vi "SR_M-Gen_Mission_annotations.vi"(10 "Op Index":i32=-1, 11 "Mission In":T1[](array[typedef]) {"GPS Longitude" format="%.6g"; "GPS Latitude" format="%.6g"}) -> (1 "Mission Path":cluster{dbl[], dbl[]}, 2 "Mission Annotation":T2(array[cluster]), 3 "Mission Out":T1[](array[typedef]) {"GPS Longitude" format="%.6g"; "GPS Latitude" format="%.6g"})   [LabVIEW 2015, in "Shore Library.lvlib"]
uses:
  Shore Library.lvlib
  RDS Mission Controller Actor/MissionOp.ctl
  RDS Mission Controller Actor/RDS Mission Controller Actor.lvlib
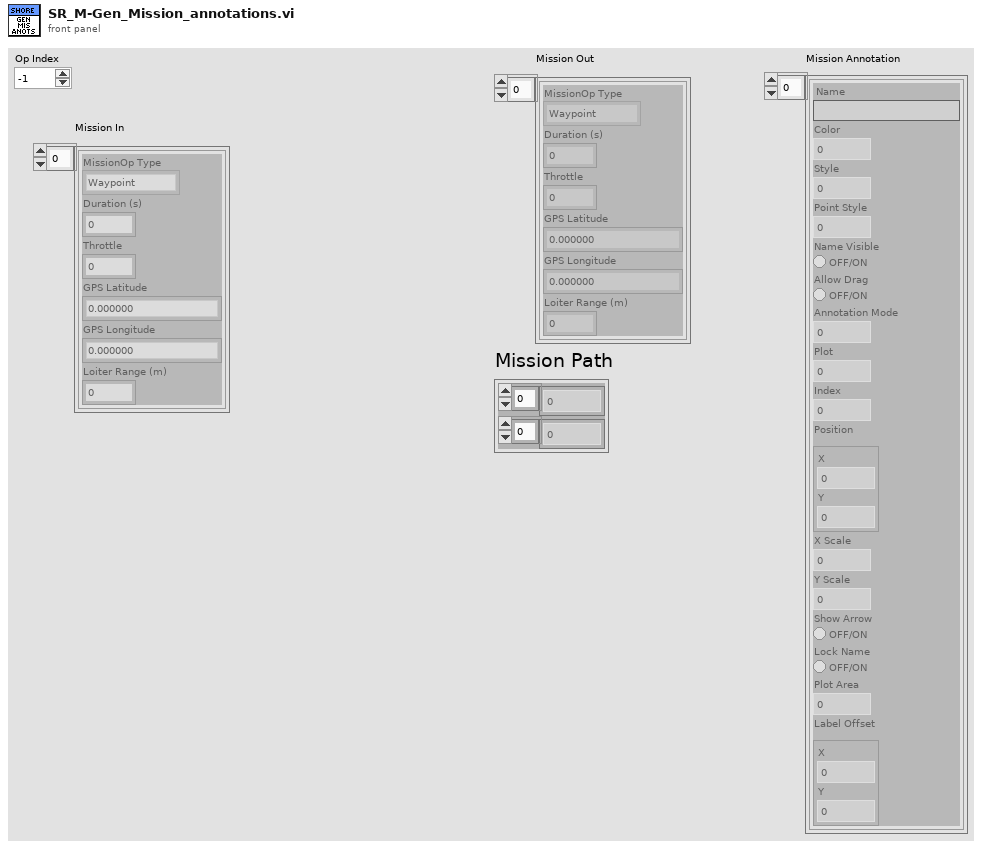
[diagram p1: front panel]
types:
  T1 = typedef "RDS Mission Controller Actor.lvlib/MissionOp.ctl" = cluster{"MissionOp Type":enum16{"Waypoint", "Loiter", "Wait", "Deploy AIP", "Stow AIP"}, "Duration (s)":u16, "Throttle":i16, "GPS Latitude":dbl, "GPS Longitude":dbl, "Loiter Range (m)":u16}
  T2 = cluster{"Name":string, "Color":u32, "Style":u8, "Point Style":u8, "Name Visible":bool, "Allow Drag":bool, "Annotation Mode":u32, "Plot":i32, "Index":i32, "Position":cluster{"X":dbl, "Y":dbl}, "X Scale":u32, "Y Scale":u32, "Show Arrow":bool, "Lock Name":bool, "Plot Area":i32, "Label Offset":cluster{"X":dbl, "Y":dbl}}[]
  T3 = cluster{"Name":string, "Color":u32, "Style":u8, "Point Style":u8, "Name Visible":bool, "Allow Drag":bool, "Annotation Mode":u32, "Plot":i32, "Index":i32, "Position":cluster{"X":dbl, "Y":dbl}, "X Scale":u32, "Y Scale":u32, "Show Arrow":bool, "Lock Name":bool, "Plot Area":i32, "Label Offset":cluster{"X":dbl, "Y":dbl}}
  T4 = enum16{"Waypoint", "Loiter", "Wait", "Deploy AIP", "Stow AIP"}
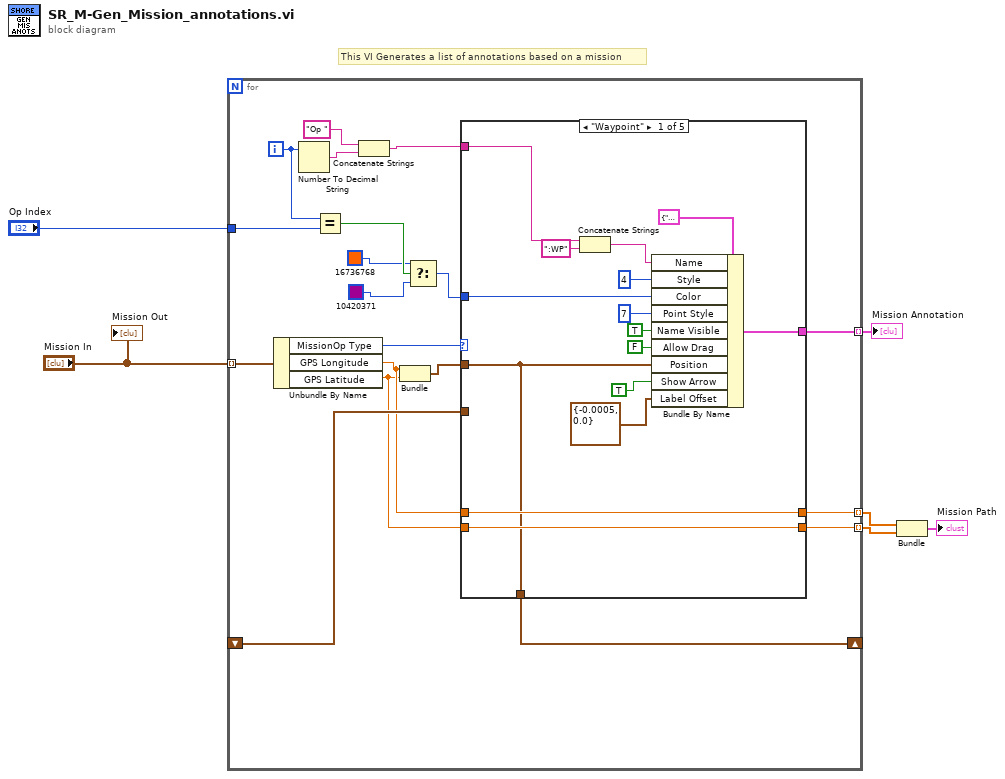
[diagram p0: block diagram]
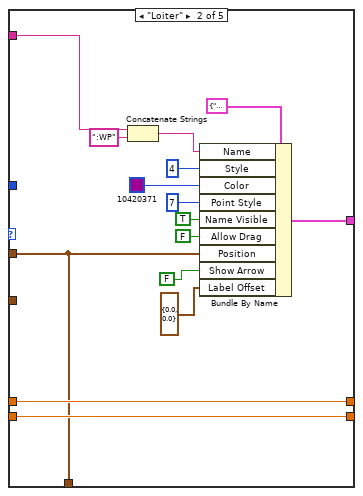
[diagram p2: hidden frame]
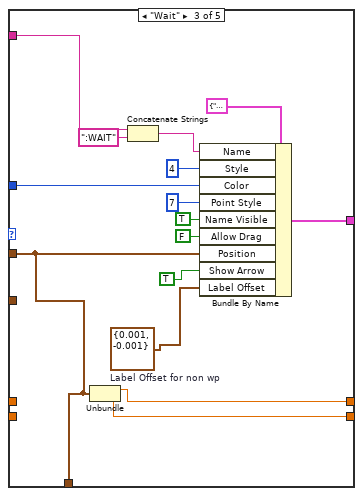
[diagram p3: hidden frame]
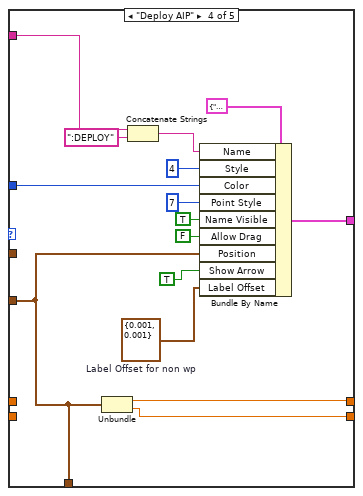
[diagram p4: hidden frame]
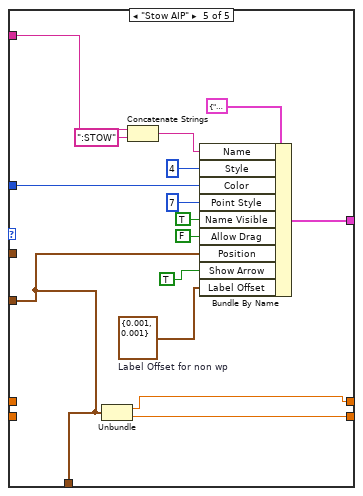
[diagram p5: hidden frame]
diagram:
  # "This VI Generates a list of annotations based on a mission"
  n1 = for {
    tunnel: "Mission In" -> [w20] mode=indexing
    tunnel: [w21] -> w5 mode=indexing
    shift-right: [w7] -> _
    shift-left: _ -> [w19]
    tunnel: "Op Index" -> [w17]
    tunnel: [w10] -> w3 mode=indexing
    tunnel: [w9] -> w2 mode=indexing
    i -> [w18]
    n2 = Unbundle By Name(w20) -> ("MissionOp Type"=w25:T4, "GPS Longitude"=w12:dbl, "GPS Latitude"=w11:dbl)
    n3 = Number To Decimal String(number=w18) -> (decimal integer string=w24:string)  [unwired: 1 in]
    n4 = Equal?(x=w18, y=w17) -> (x = y?=w16:bool)
    n5 = Concatenate Strings("Op " ("string"), w24) -> (w22:string)
    n6 = Bundle("GPS Longitude"=w12, "GPS Latitude"=w11) -> (w8:cluster{"GPS Longitude":dbl, "GPS Latitude":dbl})  [unwired: 1 in]
    n7 = Select(t=u32 16736768 ("Color of Annotation Text"), s=w16, f=u32 10420371 ("Color of Annotation Text")) -> (s? t:f=w14:u32)
    n8 = case shown="\"Waypoint\"" w25 {
      tunnel: w22 -> [w32 w46 w63 w78 w93]
      tunnel: [w33 w47 w64 w79 w94] -> w21
      tunnel: w8 -> [w26 w41 w56 _ _]
      tunnel: w14 -> [w29 _ w60 w75 w90]
      tunnel: w19 -> [_ _ _ w71 w86]
      tunnel: w12 -> [w28 w43 _ _ _]
      tunnel: w11 -> [w27 w42 _ _ _]
      tunnel: [w28 w43 w58 w73 w88] -> w10
      tunnel: [w27 w42 w57 w72 w87] -> w9
      tunnel: [w26 w41 w56 w71 w86] -> w7
      frame "Waypoint" {
        n9 = Concatenate Strings(w32, ":WP" ("string")) -> (w31:string)
        n10 = Bundle By Name(cluster=T3 {"Name"="", "Color"=0, "Style"=0, "Point Style"=0, "Name Visible"=FALSE, "Allow Drag"=FALSE, "Annotation Mode"=0, "Plot"=0, "Index"=0, "Position"={"X"=0.0, "Y"=0.0}, "X Scale"=0, "Y Scale"=0, "Show Arrow"=FALSE, "Lock Name"=FALSE, "Plot Area"=0, "Label Offset"={"X"=0.0, "Y"=0.0}}, "Name"=w31, "Style"=u8 4, "Color"=w29, "Point Style"=u8 7, "Name Visible"=TRUE, "Allow Drag"=FALSE, "Position"=w26, "Show Arrow"=TRUE, "Label Offset"=cluster{"X":dbl, "Y":dbl} {"X"=-0.0005, "Y"=0.0}) -> (w33:T3)
      }
      frame "Loiter" {
        n11 = Concatenate Strings(w46, ":WP" ("string")) -> (w45:string)
        n12 = Bundle By Name(cluster=T3 {"Name"="", "Color"=0, "Style"=0, "Point Style"=0, "Name Visible"=FALSE, "Allow Drag"=FALSE, "Annotation Mode"=0, "Plot"=0, "Index"=0, "Position"={"X"=0.0, "Y"=0.0}, "X Scale"=0, "Y Scale"=0, "Show Arrow"=FALSE, "Lock Name"=FALSE, "Plot Area"=0, "Label Offset"={"X"=0.0, "Y"=0.0}}, "Name"=w45, "Style"=u8 4, "Color"=u32 10420371 ("Color of Annotation Text"), "Point Style"=u8 7, "Name Visible"=TRUE, "Allow Drag"=FALSE, "Position"=w41, "Show Arrow"=FALSE, "Label Offset"=cluster{"X":dbl, "Y":dbl} {"X"=0.0, "Y"=0.0}) -> (w47:T3)
      }
      frame "Wait" {
        w59 = cluster{"X":dbl, "Y":dbl} {"X"=0.001, "Y"=-0.001}  # Label Offset for non wp
        n13 = Unbundle(w56) -> ("GPS Longitude"=w58:dbl, "GPS Latitude"=w57:dbl)
        n14 = Concatenate Strings(w63, ":WAIT" ("string")) -> (w62:string)
        n15 = Bundle By Name(cluster=T3 {"Name"="", "Color"=0, "Style"=0, "Point Style"=0, "Name Visible"=FALSE, "Allow Drag"=FALSE, "Annotation Mode"=0, "Plot"=0, "Index"=0, "Position"={"X"=0.0, "Y"=0.0}, "X Scale"=0, "Y Scale"=0, "Show Arrow"=FALSE, "Lock Name"=FALSE, "Plot Area"=0, "Label Offset"={"X"=0.0, "Y"=0.0}}, "Name"=w62, "Style"=u8 4, "Color"=w60, "Point Style"=u8 7, "Name Visible"=TRUE, "Allow Drag"=FALSE, "Position"=w56, "Show Arrow"=TRUE, "Label Offset"=w59) -> (w64:T3)
      }
      frame "Deploy AIP" {
        w74 = cluster{"X":dbl, "Y":dbl} {"X"=0.001, "Y"=0.001}  # Label Offset for non wp
        n16 = Unbundle(w71) -> ("GPS Longitude"=w73:dbl, "GPS Latitude"=w72:dbl)
        n17 = Concatenate Strings(w78, ":DEPLOY" ("string")) -> (w77:string)
        n18 = Bundle By Name(cluster=T3 {"Name"="", "Color"=0, "Style"=0, "Point Style"=0, "Name Visible"=FALSE, "Allow Drag"=FALSE, "Annotation Mode"=0, "Plot"=0, "Index"=0, "Position"={"X"=0.0, "Y"=0.0}, "X Scale"=0, "Y Scale"=0, "Show Arrow"=FALSE, "Lock Name"=FALSE, "Plot Area"=0, "Label Offset"={"X"=0.0, "Y"=0.0}}, "Name"=w77, "Style"=u8 4, "Color"=w75, "Point Style"=u8 7, "Name Visible"=TRUE, "Allow Drag"=FALSE, "Position"=w71, "Show Arrow"=TRUE, "Label Offset"=w74) -> (w79:T3)
      }
      frame "Stow AIP" {
        w89 = cluster{"X":dbl, "Y":dbl} {"X"=0.001, "Y"=0.001}  # Label Offset for non wp
        n19 = Unbundle(w86) -> ("GPS Longitude"=w88:dbl, "GPS Latitude"=w87:dbl)
        n20 = Concatenate Strings(w93, ":STOW" ("string")) -> (w92:string)
        n21 = Bundle By Name(cluster=T3 {"Name"="", "Color"=0, "Style"=0, "Point Style"=0, "Name Visible"=FALSE, "Allow Drag"=FALSE, "Annotation Mode"=0, "Plot"=0, "Index"=0, "Position"={"X"=0.0, "Y"=0.0}, "X Scale"=0, "Y Scale"=0, "Show Arrow"=FALSE, "Lock Name"=FALSE, "Plot Area"=0, "Label Offset"={"X"=0.0, "Y"=0.0}}, "Name"=w92, "Style"=u8 4, "Color"=w90, "Point Style"=u8 7, "Name Visible"=TRUE, "Allow Drag"=FALSE, "Position"=w86, "Show Arrow"=TRUE, "Label Offset"=w89) -> (w94:T3)
      }
    }
  }
  "Mission Annotation" <- w5
  n22 = Bundle(w3, w2) -> (→"Mission Path":cluster{dbl[], dbl[]})  [unwired: 1 in]
  "Mission Out" <- "Mission In"
